vi "Launcher View.vi"(8 "error in (no error)":errorcluster, 11 "[V] Main UI in":refnum<class "[V] Main UI.lvclass">) -> (0 "error out":errorcluster, 3 "[V] Main UI out":refnum<class "[V] Main UI.lvclass">)   [LabVIEW 2020, in "[V] Main UI.lvlib" / "[V] Main UI.lvclass"]
uses:
  [V] Main UI.lvclass
  Table View/Table View/Table View.lvclass
  C:/Program Files (x86)/National Instruments/LabVIEW 2020/vi.lib/ActorFramework/Actor/Actor.lvclass
  [V]Waveform Display/[V]Waveform Display/[V]Waveform Display.lvclass
  System Tree View/System Tree View/[V]System Tree View.lvclass
  [V] Main UI.lvclass/[V] Main UI.ctl
  Depden On/Abstruct View/Abstruct View/Abstruct View.lvclass/Abstruct View.ctl
  <vilib>/ActorFramework/Message Enqueuer/Message Enqueuer.lvclass/Message Enqueuer.ctl
  Depden On/Abstruct View/Abstruct View/Data Accessors/Write Panel Ref 1.vi
  <vilib>/ActorFramework/Message Enqueuer/Enqueue.vi
  Depden On/Abstruct View/Abstruct View Messages/Insert Panel Msg/Insert Panel Msg.lvclass
  C:/Program Files (x86)/National Instruments/LabVIEW 2020/vi.lib/ActorFramework/Message/Message.lvclass
  <vilib>/ActorFramework/Message Priority Queue/Priority Enqueue.vi
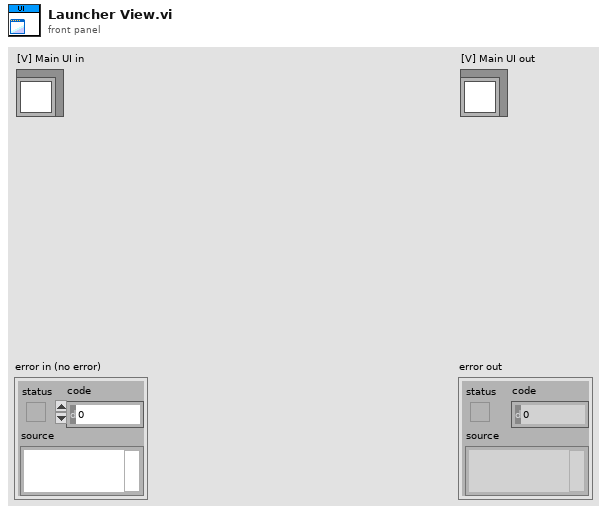
[diagram p1: front panel]
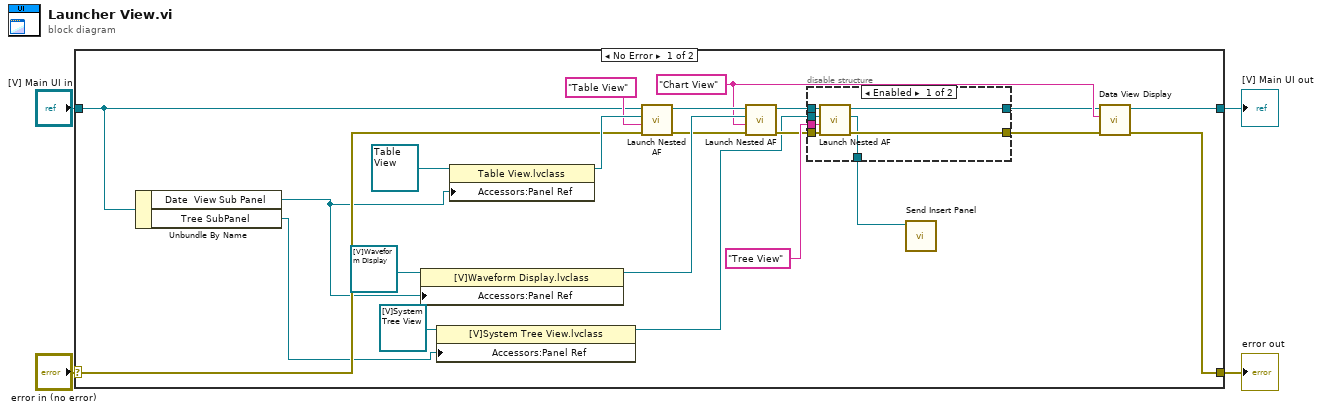
[diagram p0: block diagram]
diagram:
  n1 = case shown="No Error" "error in (no error)" {
    selector: "error in (no error)" -> [w19 w36]
    tunnel: [w15 w36] -> w3
    tunnel: [w17 w35] -> w1
    tunnel: "[V] Main UI in" -> [w18 w35]
    frame No Error {
      w16 = "Chart View" ("name")
      n2 = Unbundle By Name(w18) -> ("Date  View Sub Panel"=w13:refnum<vi>, "Tree SubPanel"=w7:refnum<vi>)
      n3 = property class="[V]Waveform Display.lvclass"(reference=refnum<class "[V]Waveform Display.lvclass"> refnum ("[V]Waveform Display.lvlib:[V]Waveform Display.lvclass"), "Accessors:Panel Ref"=w13) -> (reference out=w21:refnum<class "[V]Waveform Display.lvclass">)  [unwired: 1 in, 1 out]
      n4 = property class="[V]System Tree View.lvclass"(reference=refnum<class "[V]System Tree View.lvclass"> refnum ("[V]System Tree View.lvlib:[V]System Tree View.lvclass"), "Accessors:Panel Ref"=w7) -> (reference out=w6:refnum<class "[V]System Tree View.lvclass">)  [unwired: 1 in, 1 out]
      n5 = property class="Table View.lvclass"(reference=refnum<class "Table View.lvclass"> refnum ("[V]Table View.lvlib:Table View.lvclass"), "Accessors:Panel Ref"=w13) -> (reference out=w24:refnum<class "Table View.lvclass">)  [unwired: 1 in, 1 out]
      n6 = call "Launch Nested AF.vi"("error in (no error)"=w19, "name"="Table View", "Nested Actor"=w24, "[V] Main UI in"=w18) -> ("error out"=w20:errorcluster, "[V] Main UI out"=w22:refnum<class "[V] Main UI.lvclass">)  [unwired: 5 in, 1 out]
      n7 = call "Launch Nested AF.vi"("error in (no error)"=w20, "name"=w16, "Nested Actor"=w21, "[V] Main UI in"=w22) -> ("error out"=w10:errorcluster, "[V] Main UI out"=w12:refnum<class "[V] Main UI.lvclass">)  [unwired: 5 in, 1 out]
      n8 = disable-structure shown="Enabled" {
        disable-tunnel: w12 -> [w33 w34]
        disable-tunnel: "Tree View" ("name") -> [w32 _]
        disable-tunnel: w10 -> [w31 _]
        disable-tunnel: [w30 _] -> w9
        disable-tunnel: [w29 w34] -> w8
        disable-tunnel: w6 -> [w28 _]
        disable-tunnel: [w27 _] -> w5
        frame Enabled {
          n9 = call "Launch Nested AF.vi"("error in (no error)"=w31, "name"=w32, "Nested Actor"=w28, "[V] Main UI in"=w33) -> ("error out"=w30:errorcluster, "Enqueuer"=w27:refnum<class "Message Enqueuer.lvclass">, "[V] Main UI out"=w29:refnum<class "[V] Main UI.lvclass">)  [unwired: 5 in]
        }
        frame Disabled {
        }
      }
      n10 = call "Send Insert Panel.vi"("Message Enqueuer"=w5) -> ()  [unwired: 9 in, 2 out]
      n11 = call "Data View Display.vi"("error in (no error)"=w9, "Name"=w16, "[V] Main UI in"=w8) -> ("error out"=w15:errorcluster, "[V] Main UI out"=w17:refnum<class "[V] Main UI.lvclass">)  [unwired: 7 in]
    }
    frame Error {
    }
  }
  "error out" <- w3
  "[V] Main UI out" <- w1
